vi "WhetherInner.vi"(1 "Error permitted":dbl, 2 "JudgePoint":dbl[](array[numeric]), 3 "InputPolygon":dbl[][](array[numeric])) -> (0 "Point inside?":bool)   [LabVIEW 2013]
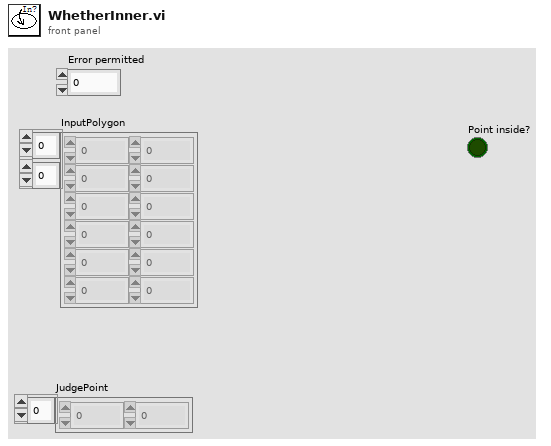
[diagram p1: front panel]
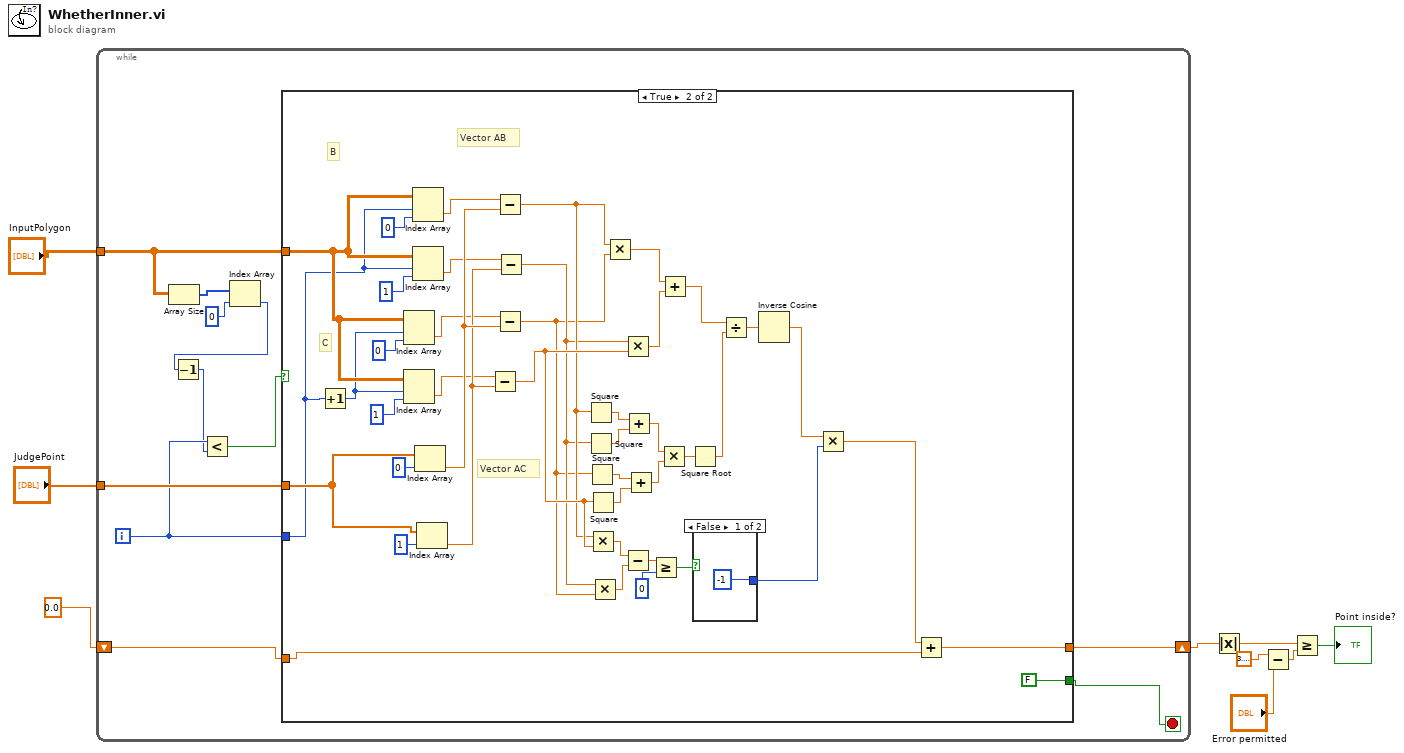
[diagram p0: block diagram]
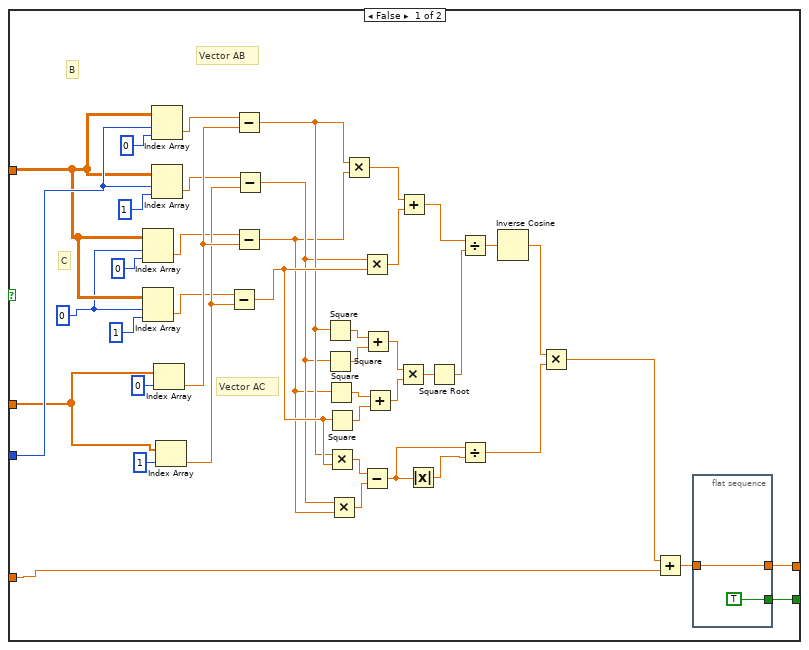
[diagram p2: hidden frame]
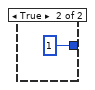
[diagram p3: hidden frame]
diagram:
  n1 = while {
    tunnel: "InputPolygon" -> [w19]
    tunnel: "JudgePoint" -> [w20]
    shift-right: [w11] -> w2
    shift-left: 0.0 -> [w12]
    i -> [w16]
    stop <- w10 stop-if-true
    n2 = Array Size(array=w19) -> (size(s)=w18:i32[])
    n3 = Index Array(array=w18, index=0) -> (element=w15:i32)
    n4 = Decrement(x=w15) -> (x-1=w14:i32)
    n5 = Less?(x=w16, y=w14) -> (x < y?=w13:bool)
    n6 = case shown="True" w13 {
      tunnel: w19 -> [w25 w101]
      tunnel: w20 -> [w26 w104]
      tunnel: w16 -> [w27 w99]
      tunnel: w12 -> [w28 w73]
      tunnel: [w22 w71] -> w11
      tunnel: [w21 FALSE] -> w10
      frame False {
        w24 = 0
        # "Vector AC"
        # "C"
        # "B"
        # "Vector AB"
        n7 = Index Array(array=w25, index (row)=w24, index (col)=0 ("disabled index (col)")) -> (element=w54:dbl)
        n8 = Index Array(array=w25, index (row)=w24, index (col)=1 ("disabled index (col)")) -> (element=w52:dbl)
        n9 = Index Array(array=w25, index (row)=w27, index (col)=0 ("disabled index (col)")) -> (element=w55:dbl)
        n10 = Index Array(array=w25, index (row)=w27, index (col)=1 ("disabled index (col)")) -> (element=w53:dbl)
        n11 = Index Array(array=w26, index=0) -> (element=w57:dbl)
        n12 = Index Array(array=w26, index=1) -> (element=w56:dbl)
        n13 = Subtract(x=w52, y=w56) -> (x-y=w39:dbl)
        n14 = Subtract(x=w55, y=w57) -> (x-y=w38:dbl)
        n15 = Subtract(x=w54, y=w57) -> (x-y=w36:dbl)
        n16 = Subtract(x=w53, y=w56) -> (x-y=w37:dbl)
        n17 = Square(x=w38) -> (x^2=w49:dbl)
        n18 = Square(x=w37) -> (x^2=w48:dbl)
        n19 = Square(x=w36) -> (x^2=w47:dbl)
        n20 = Square(x=w39) -> (x^2=w46:dbl)
        n21 = Multiply(x=w38, y=w39) -> (x*y=w35:dbl)
        n22 = Multiply(x=w37, y=w36) -> (x*y=w34:dbl)
        n23 = Multiply(x=w38, y=w36) -> (x*y=w51:dbl)
        n24 = Multiply(x=w37, y=w39) -> (x*y=w50:dbl)
        n25 = Subtract(x=w35, y=w34) -> (x-y=w33:dbl)
        n26 = Add(x=w49, y=w48) -> (x+y=w44:dbl)
        n27 = Add(x=w47, y=w46) -> (x+y=w45:dbl)
        n28 = Multiply(x=w44, y=w45) -> (x*y=w43:dbl)
        n29 = Add(x=w51, y=w50) -> (x+y=w42:dbl)
        n30 = Absolute Value(x=w33) -> (abs(x)=w32:dbl)
        n31 = Square Root(x=w43) -> (sqrt(x)=w41:dbl)
        n32 = Divide(x=w42, y=w41) -> (x/y=w40:dbl)
        n33 = Divide(x=w33, y=w32) -> (x/y=w30:dbl)
        n34 = Inverse Cosine(1:w40) -> (0:w31:dbl)
        n35 = Multiply(x=w31, y=w30) -> (x*y=w29:dbl)
        n36 = Add(x=w29, y=w28) -> (x+y=w23:dbl)
        n37 = flat-sequence {
          tunnel: w23 -> [w65]
          tunnel: [w65] -> w22
          tunnel: [TRUE] -> w21
          frame #0 {
          }
        }
      }
      frame True {
        # "Vector AC"
        # "C"
        # "B"
        # "Vector AB"
        n38 = Increment(x=w99) -> (x+1=w100:i32)
        n39 = Index Array(array=w101, index (row)=w100, index (col)=0 ("disabled index (col)")) -> (element=w95:dbl)
        n40 = Index Array(array=w101, index (row)=w100, index (col)=1 ("disabled index (col)")) -> (element=w93:dbl)
        n41 = Index Array(array=w101, index (row)=w99, index (col)=0 ("disabled index (col)")) -> (element=w96:dbl)
        n42 = Index Array(array=w101, index (row)=w99, index (col)=1 ("disabled index (col)")) -> (element=w94:dbl)
        n43 = Index Array(array=w104, index=0) -> (element=w98:dbl)
        n44 = Index Array(array=w104, index=1) -> (element=w97:dbl)
        n45 = Subtract(x=w93, y=w97) -> (x-y=w80:dbl)
        n46 = Subtract(x=w96, y=w98) -> (x-y=w79:dbl)
        n47 = Subtract(x=w95, y=w98) -> (x-y=w77:dbl)
        n48 = Subtract(x=w94, y=w97) -> (x-y=w78:dbl)
        n49 = Square(x=w79) -> (x^2=w90:dbl)
        n50 = Square(x=w78) -> (x^2=w89:dbl)
        n51 = Square(x=w77) -> (x^2=w88:dbl)
        n52 = Square(x=w80) -> (x^2=w87:dbl)
        n53 = Multiply(x=w79, y=w80) -> (x*y=w76:dbl)
        n54 = Multiply(x=w78, y=w77) -> (x*y=w75:dbl)
        n55 = Multiply(x=w79, y=w77) -> (x*y=w92:dbl)
        n56 = Multiply(x=w78, y=w80) -> (x*y=w91:dbl)
        n57 = Subtract(x=w76, y=w75) -> (x-y=w69:dbl)
        n58 = Add(x=w90, y=w89) -> (x+y=w85:dbl)
        n59 = Add(x=w88, y=w87) -> (x+y=w86:dbl)
        n60 = Greater Or Equal?(x=w69, y=0) -> (x >= y?=w67:bool)
        n61 = Multiply(x=w85, y=w86) -> (x*y=w84:dbl)
        n62 = Add(x=w92, y=w91) -> (x+y=w83:dbl)
        n63 = Square Root(x=w84) -> (sqrt(x)=w82:dbl)
        n64 = case shown="False" w67 {
          tunnel: [-1 1] -> w66
          frame False {
          }
          frame True {
          }
        }
        n65 = Divide(x=w83, y=w82) -> (x/y=w81:dbl)
        n66 = Inverse Cosine(1:w81) -> (0:w74:dbl)
        n67 = Multiply(x=w74, y=w66) -> (x*y=w72:dbl)
        n68 = Add(x=w72, y=w73) -> (x+y=w71:dbl)
      }
    }
  }
  n69 = Absolute Value(x=w2) -> (abs(x)=w1:dbl)
  n70 = Subtract(x=3.141592653589793, y="Error permitted") -> (x-y=w6:dbl)
  n71 = Greater Or Equal?(x=w1, y=w6) -> (x >= y?=→"Point inside?":bool)
